vi "IPv4wPort2Bytestring.vi"(8 "error in":errorcluster, 9 "byte order (0:big-endian, network order)":T1(ring), 11 "ip address : port":string) -> (0 "error out":errorcluster, 3 "byte string":string)   [LabVIEW 2020]
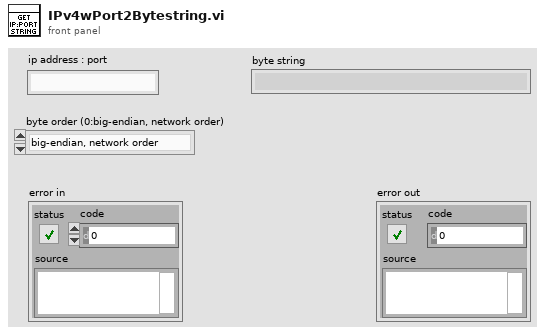
[diagram p1: front panel]
types:
  T1 = enum16{"big-endian, network order", "native, host order", "little-endian"}
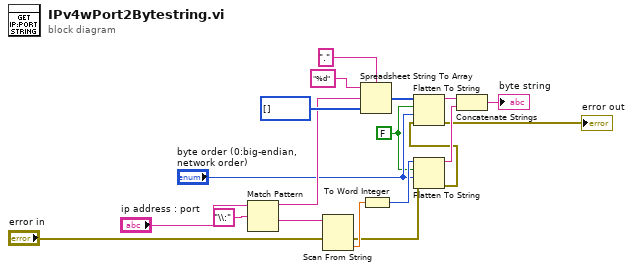
[diagram p0: block diagram]
diagram:
  w5 = FALSE ("prepend array or string size? (T)")
  n1 = Match Pattern(string="ip address : port", regular expression="\\:") -> (before substring=w12:string, after substring=w17:string)  [unwired: 1 in, 2 out]
  n2 = Scan From String(input string=w17, error in="error in") -> (error out=w3:errorcluster, output 1=w16:dbl)  [unwired: 3 in, 2 out]
  n3 = Spreadsheet String To Array(delimiter (Tab)=".", format string="%d", spreadsheet string=w12, array type (2D Dbl)=u8[] []) -> (array=w10:u8[])
  n4 = To Word Integer(number=w16) -> (16bit integer=w15:i16)
  n5 = Flatten To String(anything=w15, prepend array or string size? (T)=w5, byte order (0:big-endian, network order)="byte order (0:big-endian, network order)", error in (no error)=w3) -> (data string=w7:string, error out=w2:errorcluster)  [unwired: 1 out]
  n6 = Flatten To String(anything=w10, prepend array or string size? (T)=w5, byte order (0:big-endian, network order)="byte order (0:big-endian, network order)", error in (no error)=w2) -> (data string=w8:string, error out=→"error out":errorcluster)  [unwired: 1 out]
  n7 = Concatenate Strings(w8, w7) -> (→"byte string":string)
